vi "FloatWsignConverter.vi"(11 "Zero Lower Limit":dbl format="%.2g") -> (3 "String":string)   [LabVIEW 2016]
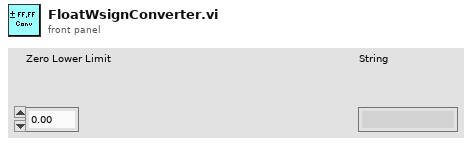
[diagram p1: front panel]
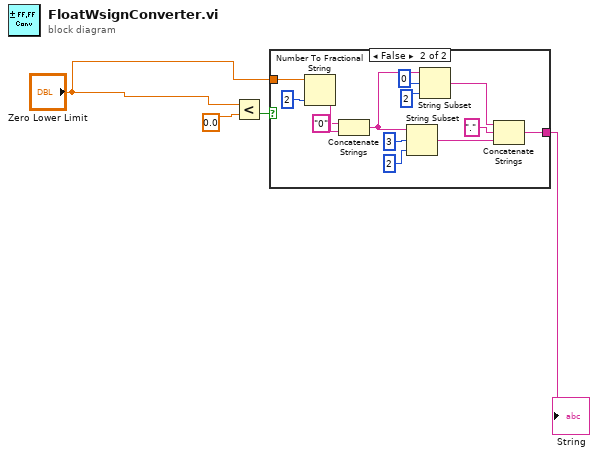
[diagram p0: block diagram]
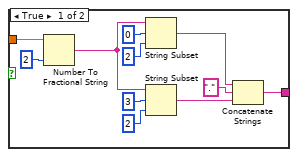
[diagram p2: hidden frame]
diagram:
  n1 = Less?(x="Zero Lower Limit", y=0.0) -> (x < y?=w2:bool)
  n2 = case shown="False" w2 {
    tunnel: "Zero Lower Limit" -> [w7 w20]
    tunnel: [w5 w19] -> w1
    frame True {
      n3 = Number To Fractional String(number=w7, precision (6)=i16 2) -> (F-format string=w6:string)  [unwired: 2 in]
      n4 = String Subset(string=w6, offset (0)=i16 0 ("precision (6)"), length (rest)=i16 2 ("precision (6)")) -> (substring=w11:string)
      n5 = String Subset(string=w6, offset (0)=i16 3 ("precision (6)"), length (rest)=i16 2 ("precision (6)")) -> (substring=w10:string)
      n6 = Concatenate Strings(w11, "." ("string"), w10) -> (w5:string)
    }
    frame False {
      n7 = Number To Fractional String(number=w20, precision (6)=i16 2) -> (F-format string=w18:string)  [unwired: 2 in]
      n8 = Concatenate Strings("0" ("string"), w18) -> (w16:string)
      n9 = String Subset(string=w16, offset (0)=i16 3 ("precision (6)"), length (rest)=i16 2 ("precision (6)")) -> (substring=w23:string)
      n10 = String Subset(string=w16, offset (0)=i16 0 ("precision (6)"), length (rest)=i16 2 ("precision (6)")) -> (substring=w24:string)
      n11 = Concatenate Strings(w24, "." ("string"), w23) -> (w19:string)
    }
  }
  "String" <- w1
